vi "Interpolate.vi"(8 "Angles":dbl[](array[numeric]), 9 "DesiredAngle":dbl, 10 "Values":dbl[](array[numeric]), 11 "Indexes":dbl[](array[numeric])) -> (3 "InterpolatedValue":dbl)   [LabVIEW 2011, in "LinearInterpolation.lvclass"]
doc: "For a pair of indexes, it determines the line between the two data points to calculate the value at the desired angle.\n\nNote: code only works if angle values do not exceed 360 degrees"
uses:
  LinearInterpolation.lvclass
  <vilib>/Analysis/NI_AALPro.lvlib
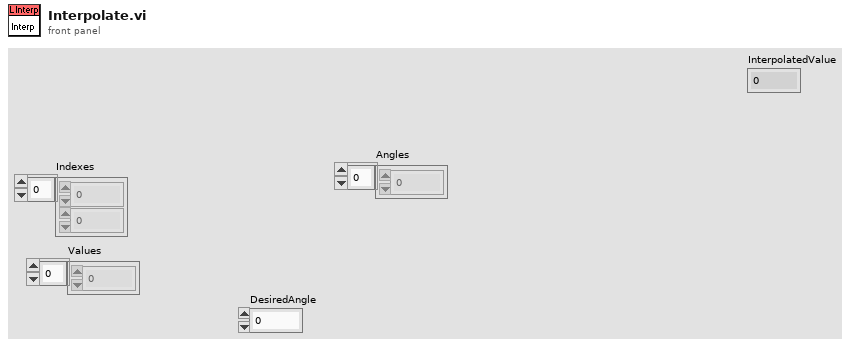
[diagram p1: front panel]
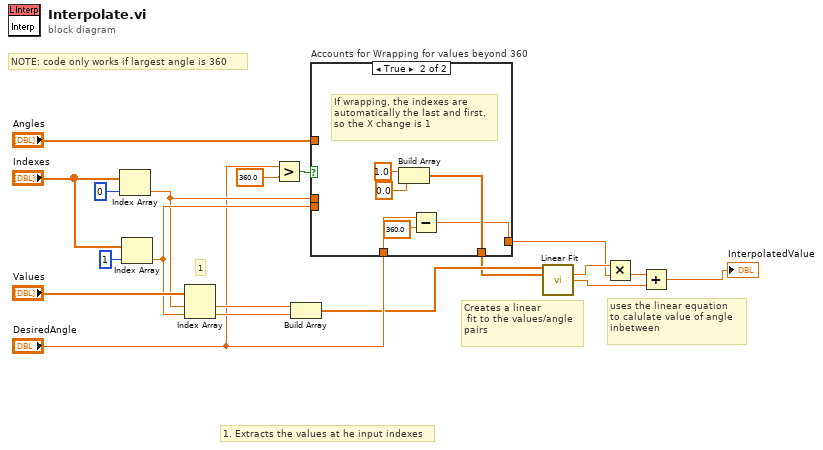
[diagram p0: block diagram]
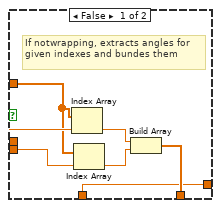
[diagram p2: hidden frame]
diagram:
  # "uses the linear equation\nto calulate value of angle \ninbetween"
  # "Creates a linear\n fit to the values/angle\npairs"
  # "NOTE: code only works if largest angle is 360"
  # "1. Extracts the values at he input indexes"
  # "1"
  n1 = Index Array(array="Indexes", index=0) -> (element=w9:dbl)
  n2 = Index Array(array="Indexes", index=1) -> (element=w10:dbl)
  n3 = Index Array(array="Values", index #1=w9, index #2=w10) -> (element #1=w8:dbl, element #2=w7:dbl)
  n4 = Greater?(x="DesiredAngle", y=360.0 ("x")) -> (0:w5:bool)
  n5 = Build Array(w8, w7) -> (w2:dbl[])
  n6 = case "Accounts for Wrapping for values beyond 360" shown="True" w5 {
    tunnel: w10 -> [w21 _]
    tunnel: [w26 w30] -> w1
    tunnel: w9 -> [w24 _]
    tunnel: "DesiredAngle" -> [w25 w29]
    tunnel: [w25 w27] -> w11
    tunnel: "Angles" -> [w20 _]
    frame False {
      # "If notwrapping, extracts angles for\ngiven indexes and bundes them"
      n7 = Index Array(array=w20, index=w24) -> (element=w22:dbl)
      n8 = Index Array(array=w20, index=w21) -> (element=w23:dbl)
      n9 = Build Array(w22, w23) -> (w26:dbl[])
    }
    frame True {
      # "If wrapping, the indexes are\nautomatically the last and first,\nso the X change is 1"
      n10 = Build Array(1.0 ("element"), 0.0 ("element")) -> (w30:dbl[])
      n11 = Subtract(x=w29, y=360.0) -> (x-y=w27:dbl)
    }
  }
  n12 = call <vilib>:"Linear Fit.vi"("Y"=w2, "X"=w1) -> ("slope"=w19:dbl, "intercept"=w17:dbl)  [unwired: 9 in, 3 out]
  n13 = Multiply(x=w19, y=w11) -> (x*y=w18:dbl)
  n14 = Add(x=w18, y=w17) -> (x+y=→"InterpolatedValue":dbl)
